vi "SVFA Zoom FFT Spectrum (Real-Im) (1 Ch).vi"(0 "scaled signal [EU]":waveform(dbl)={"t0"=timestamp(0 s since 1904-01-01), "dt"=1e-05, "Y"=[]}, 3 "zoom settings":T2={"frequency range"={"start frequency"=1000.0, "stop frequency"=2000.0}, "window"=1, "number of lines"=400, "% overlap"=0.0} {"% overlap" min=0.0 format="%.2f"; "number of lines" min=2; "window" items=["None ", "Hanning", "Hamming", "Blackman-Harris", "Exact Blackman", "Blackman", "Flat Top", "4 Term B-Harris ", "7 Term B-Harris", "Low Sidelobe"]; "frequency range"."stop frequency" min=0.0 format="%.2f"; "frequency range"."start frequency" min=0.0 format="%.2f"}, 5 "error in (no error)":errorcluster, 7 "averaging parameters":T9={"averaging mode"=enum."No averaging", "weighting mode"=enum."Exponential", "number of averages"=10, "linear mode"=enum."One shot"} {"number of averages" min=1 step=1}, 9 "restart averaging (F)":bool) -> (11 "averaging done":bool, 12 "new spectrum available":bool, 13 "averages completed":dbl, 14 "real part [EU rms]":cluster{"f0":dbl, "df":dbl, "real part":dbl[]} {"real part" format="%.2f"; "df" format="%.2f"; "f0" format="%.2f"}, 16 "imaginary part [EU rms]":T1 {"imaginary part" format="%.2f"; "df" format="%.2f"; "f0" format="%.2f"}, 17 "unit label":string, 18 "spectrum info":T3={"channel name"="", "description"="", "x-axis units"=0, "spectral info"={"spectrum type"=enum."Power [Magnitude^2]", "linear/dB"=enum."linear", "window"=0, "window size"=0, "FFT size"=0}, "engineering units"=0, "custom label"="", "dB reference [EU]"=0.0, "peak units"=enum."rms", "weighting filter"=0, "spectral density?"=FALSE, "unit label"="", "spectrum skewed?"=FALSE, "complimentary spectrum units"=enum."none"} {"x-axis units" items=["Time (s)"=0, "Frequency-CB (Hz)"=1, "Frequency-CPB (Hz)"=1248, "Frequency-Arbitrary (Hz)"=2357, "Quefrency (s)"=2, "Revolutions (rev)"=3, "Order"=4, "Speed (RPM)"=11, "Speed (rad/s)"=21, "Index"=65535]; "weighting filter" items=["Linear", "A-weighting", "B-weighting", "C-weighting", "ITU-R 468-4", "Dolby", "CCITT", "C-message", "Wb", "Wc", "Wd", "We", "Wf", "Wh", "Wj", "Wk", "Wm", "AES17 20 kHz lowpass", "AES17 40 kHz lowpass", "AES17 20 kHz highpass", "AES17 40 kHz highpass"]; "dB reference [EU]" format="%.2f"; "engineering units" items=["custom..."=0, "V"=1, "A"=21, "C"=30, "pC"=31, "s"=32, "-"=29, "Pa"=2, "N"=20, "g"=3, "m/s^2"=4, "m/s"=5, "m"=6, "mm/s"=12, "mm"=13, "micron/s"=14, "micron"=15, "in/s^2"=7, "in/s"=8, "in"=9, "mil/s"=10, "mil"=11, "rad/s^2"=16, "rad/s"=17, "rad"=18, "deg/s^2"=26, "deg/s"=27, "deg"=28, "RPM"=22, "cycle/s^2"=23, "Hz"=24, "cycle"=25, "strain"=19]; "spectral info"."window" items=["None "=0, "Hanning"=1, "Hamming"=2, "Blackman-Harris"=3, "Exact Blackman"=4, "Blackman"=5, "Flat Top"=6, "4 Term B-Harris "=7, "7 Term B-Harris"=8, "Low Sidelobe"=9, "Force - Exponential"=10, "Gaussian"=62]}, 19 "error out":errorcluster)   [LabVIEW 2017]
doc: "Computes the zoom FFT spectrum of <B>scaled signal [EU]</B> and <B>zoom settings</B>. Zoom FFT results are returned as real part and imaginary part. Data accumulates each time this VI is called. However, it returns a new spectrum only when sufficient data accumulates. Indicators and subsequent processing should only be called when <B>new spectrum available</B> is TRUE. Wire data to the <B>scaled signal [EU]</B> input to determine the polymorphic instance to use or manually select the instance."
uses:
  <vilib>/addons/_NISVFA/_Shared subVIs/Controls/svc_Spectrum Info.ctl
  <vilib>/addons/_NISVFA/_Shared subVIs/Controls/svc_X-Axis Units.ctl
  <vilib>/addons/_NISVFA/_Shared subVIs/Controls/svc_Spectrum Type.ctl
  <vilib>/addons/_NISVFA/_Shared subVIs/Controls/svc_Engineering Units Text Ring.ctl
  <vilib>/addons/_NISVFA/_Shared subVIs/Controls/svc_Weighting Filter Text Ring.ctl
  <vilib>/addons/_NISVFA/_Shared subVIs/Controls/svc_Complimentary Spectrum Units.ctl
  <vilib>/addons/_NISVFA/_Shared subVIs/Common/svc_Get SV Channel Info.vi
  <vilib>/addons/_NISVFA/_Shared subVIs/Common/svc_Spectrum Units.vi
  <vilib>/addons/_NISVFA/_Shared subVIs/Spectrum Averaging/svfa_Reset Averaging State Info.vi
  <vilib>/addons/_NISVFA/_Shared subVIs/Spectrum Averaging/svfa_Average Array with Avg Checks (complex) No State.vi
  <vilib>/addons/_NISVFA/_Shared subVIs/Common/svc_Complex to Mag2 Array.vi
  <vilib>/addons/_NISVFA/_Shared subVIs/Spectrum Averaging/svfa_Average Array with Avg Checks (real) No State.vi
  <vilib>/addons/_NISVFA/_Shared subVIs/Spectrum Averaging/svfa_Average Array (complex) No State.vi
  <vilib>/addons/_NISVFA/_Shared subVIs/Spectrum Averaging/svfa_Average Array (real) No State.vi
  <vilib>/addons/_NISVFA/_Shared subVIs/Spectrum Averaging/svfa_No Average Array (complex).vi
  <vilib>/addons/_NISVFA/_Shared subVIs/Spectrum Averaging/svfa_Average Array (complex).vi
  <vilib>/addons/_NISVFA/_Shared subVIs/Spectrum Averaging/svfa_No Average Array (real).vi
  <vilib>/addons/_NISVFA/_Shared subVIs/Spectrum Averaging/svfa_Average Array (real).vi
  <vilib>/addons/_NISVFA/_Shared subVIs/Spectrum Averaging/svfa_Peak Hold Array.vi
  <vilib>/addons/_NISVFA/_Shared subVIs/Common/svc_Get Weighting Enum and Labels.vi
  <vilib>/addons/_NISVFA/_Shared subVIs/Common/svc_Unit Label Lexical Class.vi
  <vilib>/addons/_NISVFA/_Shared subVIs/Common/svc_Engineering Units to Unit Label.vi
  <vilib>/addons/_NISVFA/_Shared subVIs/Common/svc_Format Value (DBL).vi
  <vilib>/addons/_NISVFA/_Shared subVIs/Common/svc_Channel Info to Spectrum Info.vi
  <vilib>/addons/_NISVFA/_Shared subVIs/Common/svc_Unit Label to Engineering Units.vi
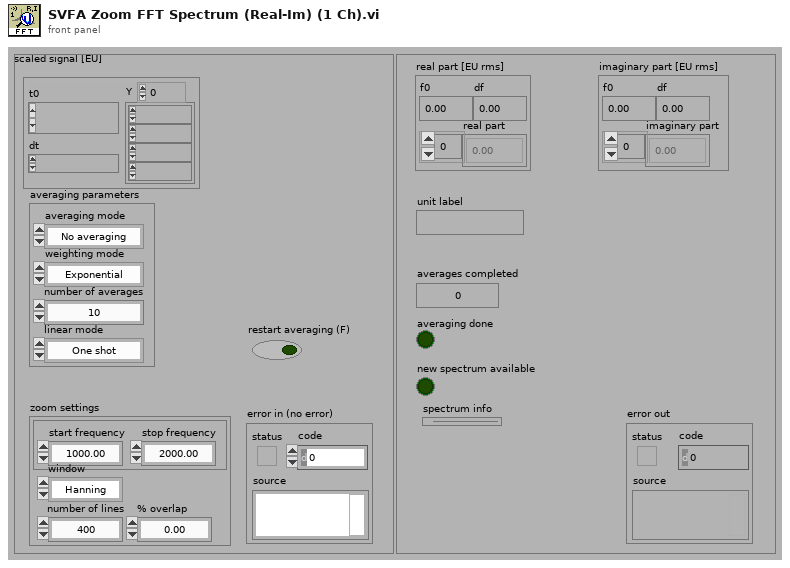
[diagram p1: front panel]
types:
  T1 = cluster{"f0":dbl, "df":dbl, "imaginary part":dbl[]}
  T2 = cluster{"frequency range":cluster{"start frequency":dbl, "stop frequency":dbl}, "window":u16, "number of lines":i32, "% overlap":dbl}
  T3 = typedef "svc_Spectrum Info.ctl" = cluster{"channel name":string, "description":string, "x-axis units":T4, "spectral info":cluster{"spectrum type":T5, "linear/dB":enum16{"linear", "dB"}, "window":u16, "window size":i32, "FFT size":i32}, "engineering units":T6, "custom label":string, "dB reference [EU]":dbl, "peak units":enum16{"rms", "peak", "peak-peak"}, "weighting filter":T7, "spectral density?":bool, "unit label":string, "spectrum skewed?":bool, "complimentary spectrum units":T8}
  T4 = typedef "svc_X-Axis Units.ctl" = u16
  T5 = typedef "svc_Spectrum Type.ctl" = enum16{"FFT Spectrum [complex]", "Amplitude [Magnitude]", "Power [Magnitude^2]", "Cross Spectrum [complex]", "Frequency Response [Complex]"}
  T6 = typedef "svc_Engineering Units Text Ring.ctl" = u16
  T7 = typedef "svc_Weighting Filter Text Ring.ctl" = u16
  T8 = typedef "svc_Complimentary Spectrum Units.ctl" = enum16{"none", "radians", "degrees", "cycles", "imaginary"}
  T9 = cluster{"averaging mode":enum16{"No averaging", "Vector averaging", "RMS averaging", "Peak hold"}, "weighting mode":enum16{"Linear", "Exponential"}, "number of averages":u32, "linear mode":enum16{"One shot", "Auto restart"}}
  T10 = enum16{"Restart processing", "Continue processing", "Skip processing"}
  T11 = enum16{"No averaging", "Vector averaging", "RMS averaging", "Peak hold"}
  T12 = cluster{"zoom settings":cluster{"center frequency":dbl, "zoom":i32, "trim":dbl}, "FFT settings":cluster{"window":enum16{"None ", "Hanning", "Hamming", "Blackman-Harris", "Exact Blackman", "Blackman", "Flat Top", "4 Term B-Harris ", "7 Term B-Harris", "Low Sidelobe"}, "window size":i32, "FFT size":i32, "%overlap":dbl}}
  T13 = cluster{"complex FFT":cdb[], "real FFT":dbl[], "f0":dbl, "df":dbl, "averages completed":dbl, "averaging parameters":cluster{"averaging mode":enum16{"No averaging", "Vector averaging", "RMS averaging", "Peak hold"}, "weighting mode":enum16{"Linear", "Exponential"}, "number of averages":u32, "linear mode":enum16{"One shot", "Auto restart"}}}
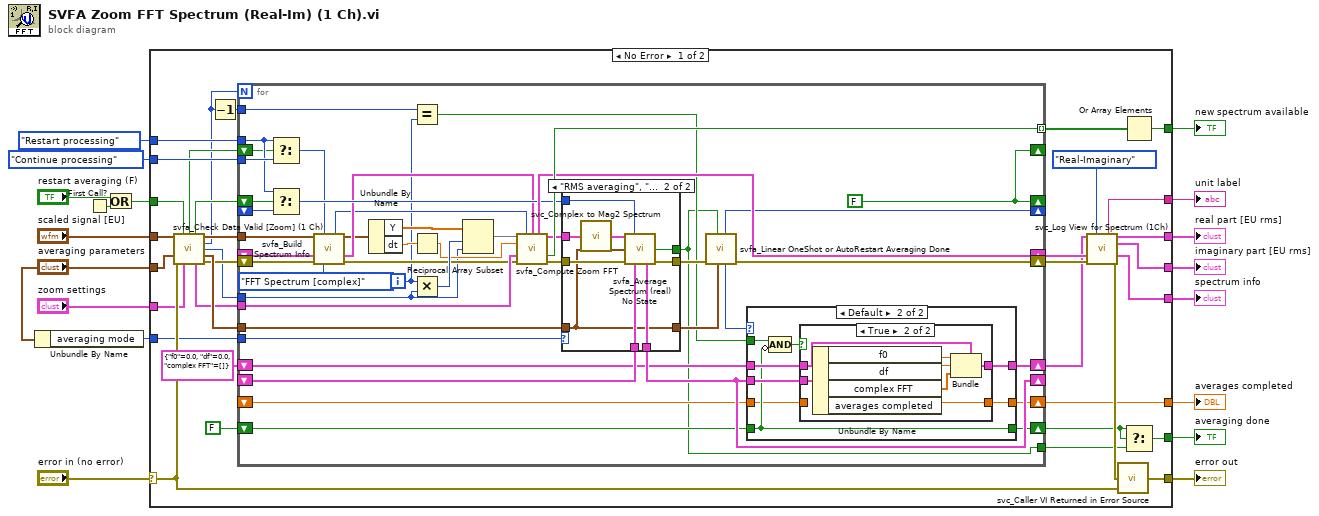
[diagram p0: block diagram]
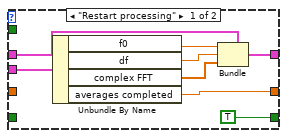
[diagram p2: hidden frame]
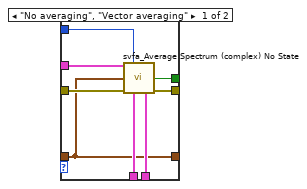
[diagram p4: hidden frame]
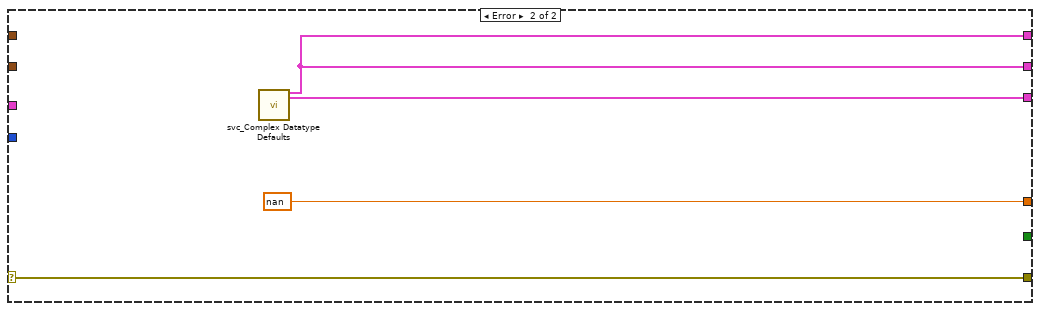
[diagram p5: hidden frame]
diagram:
  n1 = Unbundle By Name("averaging parameters") -> ("averaging mode"=w1:T11)
  n2 = First Call?() -> (First Call?: T/F=w7:bool)
  n3 = Or(x="restart averaging (F)", y=w7) -> (x .or. y?=w5:bool)
  n4 = case shown="No Error" "error in (no error)" {
    selector: "error in (no error)" -> [w42 w144]
    tunnel: w5 -> [w32 _]
    tunnel: [w20 nan ("Averaged So-far")] -> w9
    tunnel: "averaging parameters" -> [w43 _]
    tunnel: "zoom settings" -> [w41 _]
    tunnel: "scaled signal [EU]" -> [w44 _]
    tunnel: [w36 w142] -> w10
    tunnel: [w39 _] -> w13
    tunnel: [w37 w141] -> w8
    tunnel: [w38 w141] -> w12
    tunnel: [w33 _] -> w14
    tunnel: [w35 w144] -> w11
    tunnel: [w25 _] -> w18
    tunnel: T10."Restart processing" ("processing control") -> [w31 _]
    tunnel: T10."Continue processing" ("processing control") -> [w30 _]
    tunnel: w1 -> [w26 _]
    frame No Error {
      n5 = call <vilib>:"svfa_Check Data Valid [Zoom] (1 Ch).vi"("signal [V]"=w44, "restart averaging (F)"=w32, "averaging parameters"=w43, "error in (no error)"=w42, "zoom settings"=w41) -> ("reset processing"=w29:bool, "restart averaging"=w47:bool, "dup signal [V]"=w51:waveform(dbl), "iterations"=w28:i32, "maximum block size"=w34:i32, "dup averaging parameters"=w50:T9, "zoom FFT settings"=w48:T12, "error out"=w49:errorcluster)  [unwired: 3 in]
      n6 = Decrement(x=w28) -> (x-1=w27:i32)
      n7 = for {
        N: w28 -> [_]
        shift-left: _ -> [w94]
        shift-right: [w65] -> _
        tunnel: [w95] -> w40 mode=indexing
        tunnel: w48 -> [w96]
        tunnel: w51 -> [w97]
        tunnel: [w55] -> w24
        shift-right: [w93] -> w46
        shift-left: _ -> [w92]
        shift-right: [w61] -> _
        shift-left: _ -> [w88]
        tunnel: w50 -> [w91]
        shift-right: [w54] -> _
        shift-left: w47 -> [w89]
        tunnel: w34 -> [w68]
        tunnel: w31 -> [w84]
        tunnel: w30 -> [w85]
        shift-right: [w54] -> _
        shift-left: w29 -> [w82]
        tunnel: w27 -> [w70]
        tunnel: w26 -> [w67]
        shift-right: [w64] -> w23
        shift-left: cluster{"f0":dbl, "df":dbl, "complex FFT":cdb[]} {"f0"=0.0, "df"=0.0, "complex FFT"=[]} -> [w63]
        shift-right: [w59] -> w19
        shift-left: FALSE ("restart averaging") -> [w57]
        shift-right: [w60] -> w20
        shift-left: _ -> [w58]
        shift-right: [w98] -> w45
        shift-left: w49 -> [w90]
        i -> [w69]
        w54 = FALSE ("restart averaging")
        n8 = Select(t=w84, s=w82, f=w85) -> (s? t:f=w83:T10)
        n9 = Select(t=w84, s=w89, f=w88) -> (s? t:f=w87:T10)
        n10 = call <vilib>:"svfa_Build Spectrum Info.vi"("scaled signal [EU]"=w97, "processing control"=w83, "spectrum info in"=w92, "error in (no error)"=w90, "spectrum type"=svc_Spectrum_Type."FFT Spectrum [complex]") -> ("dup processing control"=w74:T10, "dup scaled signal [EU]"=w77:waveform(dbl), "spectrum info out"=w79:T3, "error out"=w72:errorcluster)  [unwired: 7 in]
        n11 = Unbundle By Name ("Get Waveform Components")(w77) -> ("Y"=w80:dbl[], "dt"=w78:dbl)
        n12 = Equal?(x=w70, y=w69) -> (x = y?=w62:bool)
        n13 = Reciprocal(x=w78) -> (1/x=w73:dbl)
        n14 = Multiply(x=w69, y=w68) -> (x*y=w86:i32)
        n15 = Array Subset(array=w80, index=w86, length=w68) -> (w71:dbl[])
        n16 = call <vilib>:"svfa_Compute Zoom FFT.vi"("x"=w71, "processing control"=w74, "spectrum info"=w79, "fs"=w73, "zoom FFT settings"=w96, "error in (no error)"=w72) -> ("spectrum info out"=w93:T3, "FFT spectrum"=w76:cluster{"f0":dbl, "df":dbl, "spectrum":cdb[]}, "spectrum ready"=w95:bool, "error out"=w75:errorcluster)  [unwired: 5 in, 1 out]
        n17 = case shown="\"RMS averaging\", \"Peak hold\"" w67 {
          tunnel: w91 -> [w124 w132]
          tunnel: [w129 w135] -> w81
          tunnel: [w128 w139] -> w55
          tunnel: w76 -> [w131 w136]
          tunnel: w75 -> [w130 w140]
          tunnel: w87 -> [w127 w137]
          tunnel: [w126 w133] -> w65
          tunnel: w94 -> [w125 w134]
          tunnel: [w124 w132] -> w66
          frame "No averaging", "Vector averaging" {
            n18 = call <vilib>:"svfa_Average Spectrum (complex) No State.vi"("spectrum"=w131, "processing control"=w127, "averaging parameters"=w124, "error in (no error)"=w130, "averaging state info in"=w125) -> ("averaging done"=w128:bool, "averaging state info out"=w126:T13, "error out"=w129:errorcluster)  [unwired: 5 in, 3 out]
          }
          frame "RMS averaging", "Peak hold" {
            n19 = call <vilib>:"svc_Complex to Mag2 Spectrum.vi"("complex spectrum"=w136) -> ("power spectrum"=w138:cluster{"f0":dbl, "df":dbl, "spectrum":dbl[]})  [unwired: 4 in]
            n20 = call <vilib>:"svfa_Average Spectrum (real) No State.vi"("spectrum"=w138, "processing control"=w137, "averaging parameters"=w132, "error in (no error)"=w140, "averaging state info in"=w134) -> ("averaging done"=w139:bool, "averaging state info out"=w133:T13, "error out"=w135:errorcluster)  [unwired: 5 in, 3 out]
          }
        }
        n21 = call <vilib>:"svfa_Linear OneShot or AutoRestart Averaging Done.vi"("averaging parameters"=w66, "averaging done"=w55, "error in (no error)"=w81) -> ("error out"=w98:errorcluster, "processing control"=w61:T10)  [unwired: 7 in]
        n22 = case shown="Default" w61 {
          tunnel: w65 -> [w103 w114]
          tunnel: [TRUE ("restart averaging") w109] -> w59
          tunnel: [w101 w113] -> w64
          tunnel: w57 -> [_ w109]
          tunnel: w62 -> [_ w112]
          tunnel: w63 -> [w100 w111]
          tunnel: [w99 w108] -> w60
          tunnel: w58 -> [_ w107]
          frame "Restart processing" {
            n23 = Unbundle By Name(w103) -> ("f0"=w106:dbl, "df"=w105:dbl, "complex FFT"=w104:cdb[], "averages completed"=w99:dbl)
            n24 = Bundle(cluster=w100, "f0"=w106, "df"=w105, "complex FFT"=w104) -> (w101:cluster{"f0":dbl, "df":dbl, "complex FFT":cdb[]})
          }
          frame Default {
            n25 = Compound Arithmetic op=AND(w112, invert w109) -> (w110:bool)
            n26 = case shown="True" w110 {
              tunnel: w114 -> [_ w120]
              tunnel: [w116 w119] -> w113
              tunnel: w111 -> [w116 w118]
              tunnel: [w115 w117] -> w108
              tunnel: w107 -> [w115 _]
              frame False {
              }
              frame True {
                n27 = Unbundle By Name(w120) -> ("f0"=w123:dbl, "df"=w122:dbl, "complex FFT"=w121:cdb[], "averages completed"=w117:dbl)
                n28 = Bundle(cluster=w118, "f0"=w123, "df"=w122, "complex FFT"=w121) -> (w119:cluster{"f0":dbl, "df":dbl, "complex FFT":cdb[]})
              }
            }
          }
        }
      }
      n29 = call <vilib>:"svc_Log View for Spectrum (1Ch).vi"("complex spectrum"=w23, "View"=enum16{"Mag-Phase", "Real-Imaginary"}."Real-Imaginary", "spectrum info in"=w46, "error in (no error)"=w45) -> ("unit label [mag or real]"=w39:string, "magnitude or real"=w38:cluster{"f0":dbl, "df":dbl, dbl[]}, "phase or imag"=w37:cluster{"f0":dbl, "df":dbl, dbl[]}, "spectrum info out"=w36:T3, "error out"=w53:errorcluster)  [unwired: 6 in, 1 out]
      n30 = call <vilib>:"svc_Caller VI Returned in Error Source.vi"("warning input to caller"=w42, "error in (no error)"=w53) -> ("error out"=w35:errorcluster)  [unwired: 3 in]
      n31 = Or Array Elements(Boolean array=w40) -> (logical OR=w33:bool)
      n32 = Select(t=w19, s=w19, f=w24) -> (s? t:f=w25:bool)
    }
    frame Error {
      n33 = call <vilib>:"svc_Complex Datatype Defaults.vi"() -> ("empty spectrum"=w141:cluster{"f0":dbl, "df":dbl, "magnitude":dbl[]}, "dead spectrum info"=w142:T3)  [unwired: 11 in, 7 out]
    }
  }
  "averages completed" <- w9
  "new spectrum available" <- w14
  "error out" <- w11
  "spectrum info" <- w10
  "unit label" <- w13
  "real part [EU rms]" <- w12
  "imaginary part [EU rms]" <- w8
  "averaging done" <- w18
